vi "解析表格数据.vi"(0 "点位信息表":string[][](table)=[["PCB1-拍照点1(Mark1)", "-73.376", "-164.238", "0.000", "-103.848", "565.620", "384.924", "377.049", "0.000", "0.000", "0.000", "0", "8", "94", "1"], ["PCB1-拍照点2(Mark2)", "-260.376", "-49.239", "0.000", "-290.450", "681.264", "384.924", "377.049", "0.000", "0.000", "0.000", "-180", "8", "94", "1"], ["拍照点3", "-73.376", "-49.239", "0.000", "-103.451", "680.618", "384.924", "377.049", "0.000", "0.000", "0.000", "0", "8", "94", "1"], ["拍照点4", "-260.376", "-164.238", "0.000", "-290.847", "566.266", "384.924", "377.049", "0.000", "0.000", "0.000", "-180", "8", "94", "1"], ["拍照点5", "-260.376", "-104.239", "0.000", "-290.640", "626.265", "384.924", "377.049", "0.000", "0.000", "0.000", "-180", "8", "94", "1"], ["拍照点6", "-240.876", "-23.738", "0.000", "-270.862", "706.698", "384.924", "377.049", "0.000", "0.000", "0.000", "90", "8", "94", "1"], ["拍照点7", "-190.876", "-23.738", "0.000", "-220.862", "706.525", "384.924", "377.049", "0.000", "0.000", "0.000", "90", "8", "94", "0"], ["拍照点8", "-142.876", "-23.738", "0.000", "-172.862", "706.359", "384.924", "377.049", "0.000", "0.000", "0.000", "90", "8", "94", "0"], ["拍照点9", "-92.876", "-23.738", "0.000", "-122.863", "706.187", "384.924", "377.049", "0.000", "0.000", "0.000", "90", "8", "94", "0"], ["拍照点10", "-73.376", "-104.239", "0.000", "-103.641", "625.619", "384.924", "377.049", "0.000", "0.000", "0.000", "0", "8", "94", "0"], ["拍照点11", "-112.876", "-169.238", "0.000", "-143.365", "560.756", "384.924", "377.049", "0.000", "0.000", "0.000", "-90", "8", "94", "0"], ["拍照点12", "-220.876", "-169.238", "0.000", "-251.364", "561.130", "384.924", "377.049", "0.000", "0.000", "0.000", "0", "8", "94", "0"], ["PCB2-拍照点1(Mark3)", "-73.376", "-164.238", "0.000", "151.457", "565.201", "384.924", "377.049", "0.000", "0.000", "-3.000", "0", "8", "94", "1"], ["PCB2-拍照点2(Mark4)", "-260.376", "-49.239", "0.000", "-35.509", "680.255", "384.924", "377.049", "0.000", "0.000", "-3.000", "-180", "8", "94", "1"], ["拍照点3", "-73.376", "-49.239", "0.000", "151.491", "680.200", "384.924", "377.049", "0.000", "0.000", "-3.000", "0", "8", "94", "1"], ["拍照点4", "-260.376", "-164.238", "0.000", "-35.543", "565.256", "384.924", "377.049", "0.000", "0.000", "-3.000", "-180", "8", "94", "1"], ["拍照点5", "-260.376", "-104.239", "0.000", "-35.525", "625.255", "384.924", "377.049", "0.000", "0.000", "-3.000", "-180", "8", "94", "1"], ["拍照点6", "-240.876", "-23.738", "0.000", "-16.001", "705.751", "384.924", "377.049", "0.000", "0.000", "-3.000", "90", "8", "94", "1"], ["拍照点7", "-190.876", "-23.738", "0.000", "33.999", "705.736", "384.924", "377.049", "0.000", "0.000", "0.000", "90", "8", "94", "0"], ["拍照点8", "-142.876", "-23.738", "0.000", "81.999", "705.722", "384.924", "377.049", "0.000", "0.000", "0.000", "90", "8", "94", "0"], ["拍照点9", "-92.876", "-23.738", "0.000", "131.999", "705.707", "384.924", "377.049", "0.000", "0.000", "0.000", "90", "8", "94", "0"], ["拍照点10", "-73.376", "-104.239", "0.000", "151.475", "625.200", "384.924", "377.049", "0.000", "0.000", "0.000", "0", "8", "94", "0"], ["拍照点11", "-112.876", "-169.238", "0.000", "111.956", "560.213", "384.924", "377.049", "0.000", "0.000", "0.000", "-90", "8", "94", "0"], ["拍照点12", "-220.876", "-169.238", "0.000", "3.956", "560.245", "384.924", "377.049", "0.000", "0.000", "0.000", "0", "8", "94", "0"]]) -> (4 "基本信息":T2, 6 "布线前甩线":string[][](table), 8 "布线点位":string[][](table), 10 "布线后甩线":string[][](table), 15 "进出线编码":cluster{"进线编码":i32, "出线编码":i32}[](array[cluster]))   [LabVIEW 2014]
uses:
  Global.vi
panel:
  out "当前线号布线轨迹示意图":T1(plugin-control)
  out "甩线后":dbl[](array[numeric])
  out "布线":dbl[](array[numeric])
  out "甩线前":dbl[](array[numeric])
  out "线号ok":bool
  out "数据正常":bool
  in  "基本信息":T2
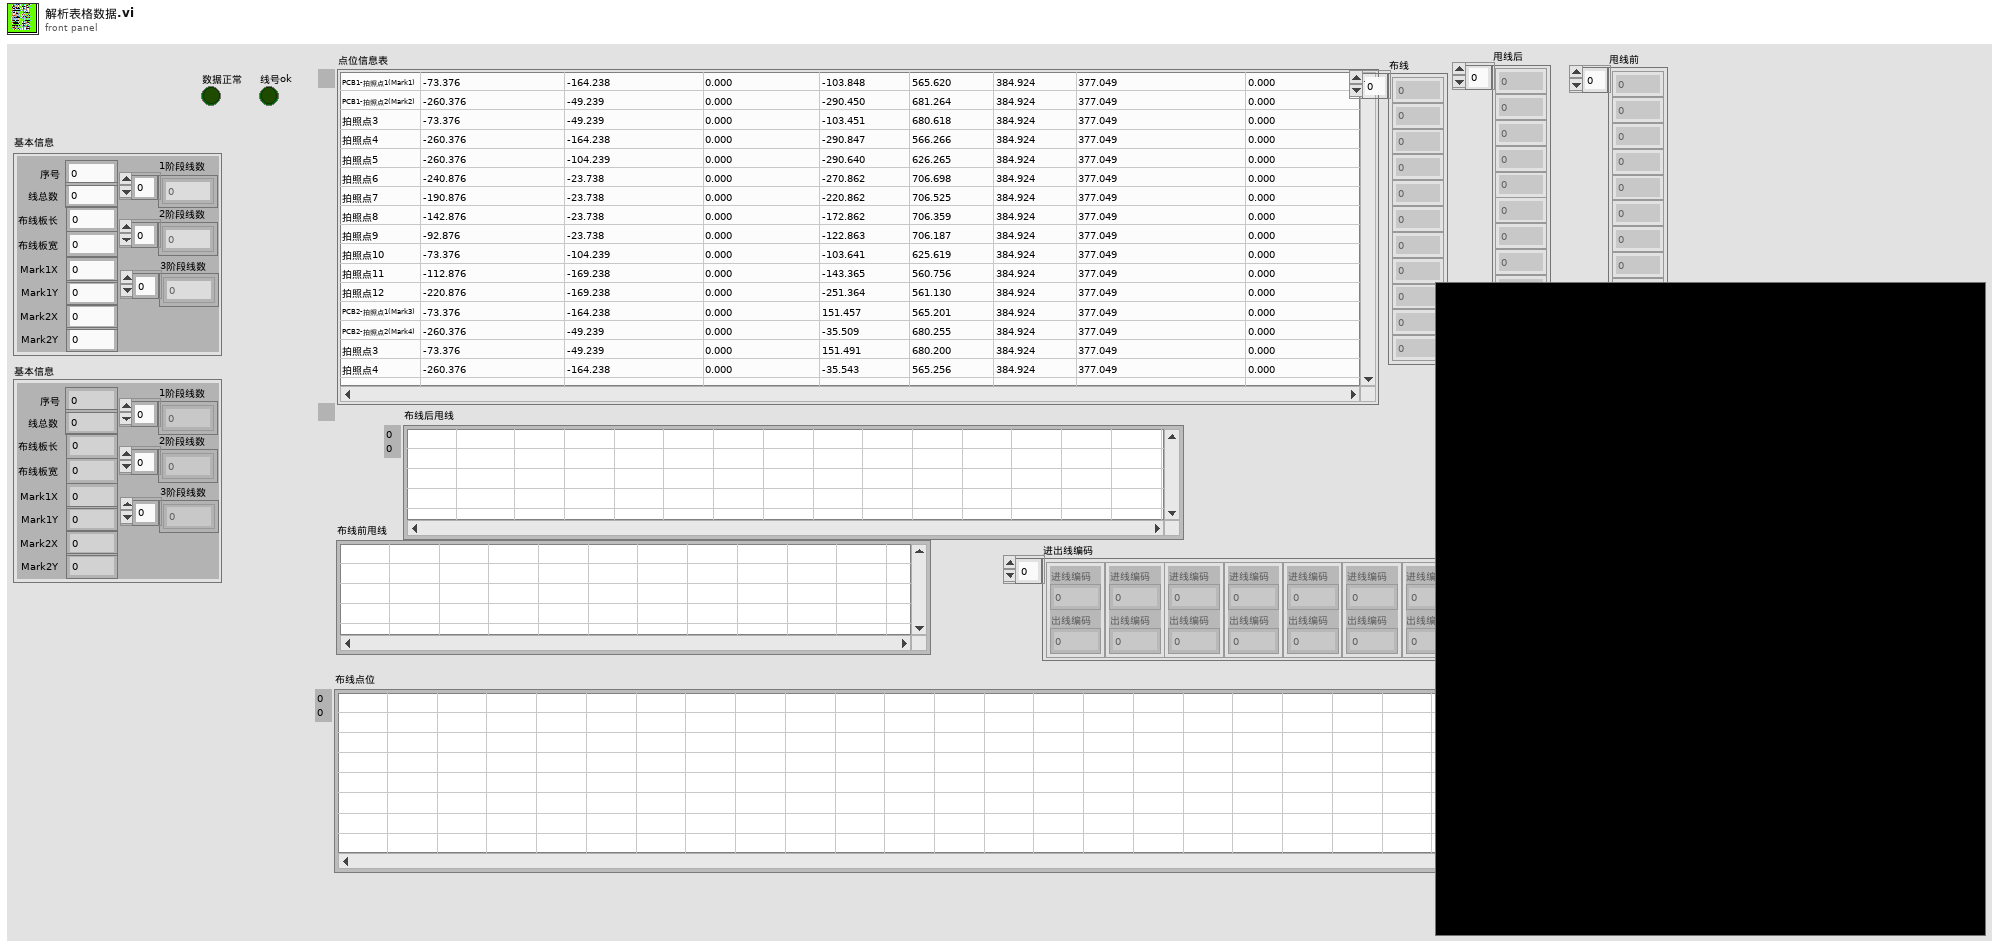
[diagram p1: front panel]
types:
  T1 = typedef "IMAQ Image.ctl" = refnum<image>
  T2 = typedef "基本信息.ctl" = cluster{"序号":dbl, "线总数":dbl, "布线板长":dbl, "布线板宽":dbl, "Mark1X":dbl, "Mark1Y":dbl, "Mark2X":dbl, "Mark2Y":dbl, "1阶段线数":dbl[], "2阶段线数":dbl[], "3阶段线数":dbl[]}
  T3 = typedef "XYPos.ctl" = cluster{"X":dbl, "Y":dbl}
  T4 = typedef "mark规格.ctl" = cluster{"X下限":dbl, "X上限":dbl, "Y下限":dbl, "Y 上限":dbl, "angle下限":dbl, "angle上限":dbl}
  T5 = cluster{"甩线补偿值":cluster{"下边":dbl, "距离上边":dbl, "左边":dbl, "右边":dbl}, "补偿甩线坐标偏移":T3, "mark点模组补偿":T3, "出线补偿值":dbl, "mark规格":T4}
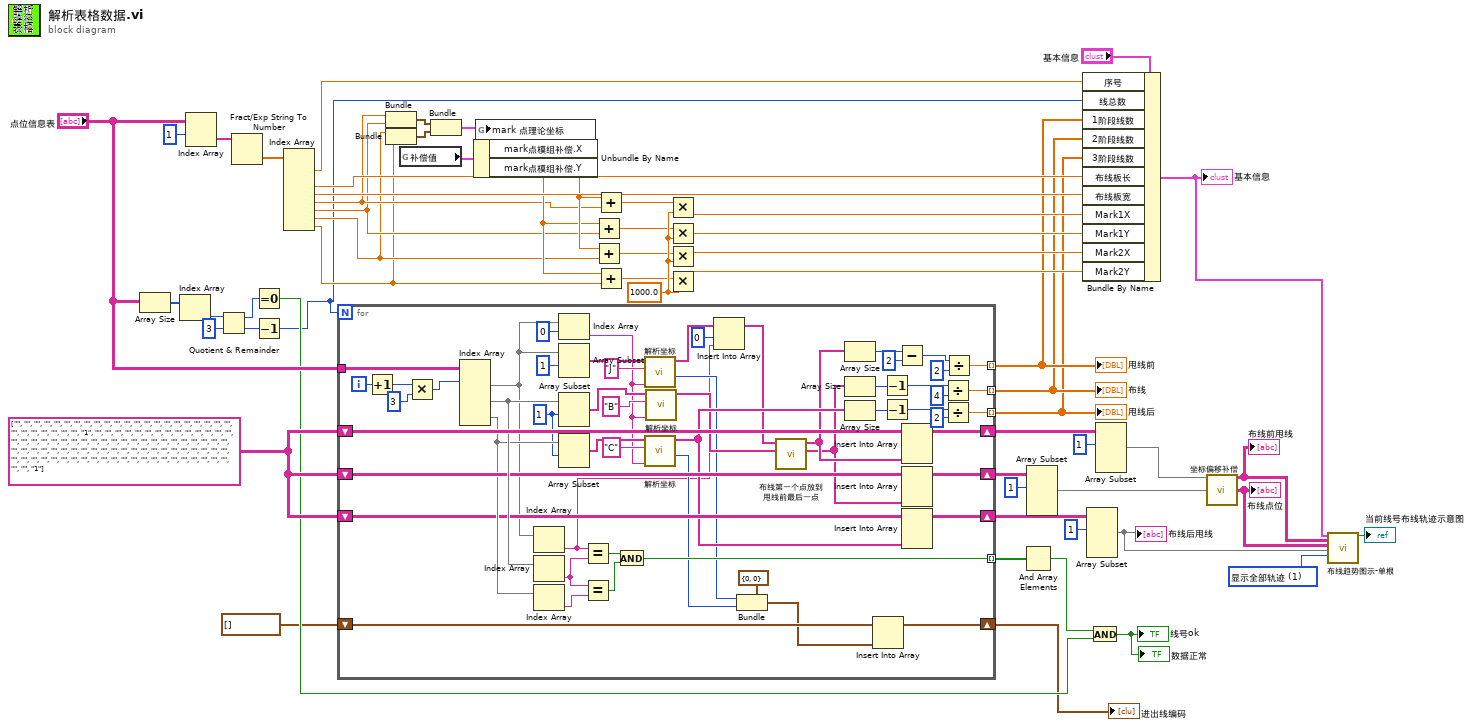
[diagram p0: block diagram]
diagram:
  w3 = u16 1 items=["显示单根轨迹", "显示全部轨迹"] ("轨迹选择")
  w23 = 1000.0 ("y")
  w50 = string[][] [["", "", "", "", "", "", "", "", "", "", "", "", "", "", "", "", "", "", "", "", "", "", "", "", "", "", "", "", "", "1", "", "", "", "", "", "", "", "", "", "", "", "", "", "", "", "", "", "", "", "", "", "", "", "", "", "", "", "", "", "", "", "", "", "", "", "", "", "", "", "", "", "", "", "", "", "", "", "", "", "", "", "", "", "", "", "", "", "", "", "", "", "", "", "", "", "", "", "", "", "", "", "", "", "", "", "", "", "", "", "", "", "", "1"]]
  n1 = Array Size(array="点位信息表") -> (size(s)=w54:i32[])
  n2 = Index Array(array=w54) -> (element=w53:i32)  [unwired: 1 in]
  n3 = Index Array(array="点位信息表", index (row)=1 ("索引 (行)")) -> (element=w56:string[])  [unwired: 1 in]
  n4 = Quotient & Remainder(x=w53, y=3) -> (x-y*floor(x/y)=w51:i32, floor(x/y)=w48:i32)
  n5 = Fract/Exp String To Number(string=w56) -> (number=w47:dbl[])  [unwired: 3 in, 1 out]
  n6 = Equal To 0?(x=w51) -> (x = 0?=w38:bool)
  n7 = Decrement(x=w48) -> (x-1=w8:i32)
  n8 = Index Array(array=w47) -> (element #1=w33:dbl, element #3=w46:dbl, element #4=w45:dbl, element #5=w16:dbl, element #6=w15:dbl, element #7=w11:dbl, element #8=w10:dbl)  [unwired: 8 in, 1 out]
  n9 = for {
    N: w8 -> [_]
    tunnel: "点位信息表" -> [w113]
    tunnel: [w104] -> w40 mode=indexing
    shift-right: [w100] -> w32
    shift-left: w50 -> [w103]
    shift-right: [w91] -> w27
    shift-left: w50 -> [w96]
    shift-right: [w90] -> w28
    shift-left: w50 -> [w89]
    tunnel: [w87] -> w36 mode=indexing
    tunnel: [w83] -> w35 mode=indexing
    tunnel: [w82] -> w34 mode=indexing
    shift-right: [w69] -> w24
    shift-left: cluster{"进线编码":i32, "出线编码":i32}[] [] -> [w71]
    i -> [w112]
    w75 = 1 ("索引")
    n10 = Increment(x=w112) -> (x+1=w109:i32)
    n11 = Multiply(x=w109, y=3) -> (x*y=w110:i32)
    n12 = Index Array(array=w113, index (row) #1=w110) -> (element #1=w78:string[], element #2=w99:string[], element #3=w94:string[])  [unwired: 5 in]
    n13 = Index Array(array=w78) -> (element=w62:string)  [unwired: 1 in]
    n14 = Index Array(array=w99) -> (element=w108:string)  [unwired: 1 in]
    n15 = Index Array(array=w94) -> (element=w107:string)  [unwired: 1 in]
    n16 = Index Array(array=w78, index=0 ("索引")) -> (element=w76:string)
    n17 = Array Subset(array=w78, index=1 ("索引")) -> (w102:string[])  [unwired: 1 in]
    n18 = Array Subset(array=w99, index=w75) -> (w97:string[])  [unwired: 1 in]
    n19 = Array Subset(array=w94, index=w75) -> (w93:string[])  [unwired: 1 in]
    n20 = Equal?(x=w62, y=w108) -> (x = y?=w106:bool)
    n21 = Equal?(x=w108, y=w107) -> (x = y?=w105:bool)
    n22 = And(x=w106, y=w105) -> (x .and. y?=w104:bool)
    n23 = call "解析坐标.vi"("线号"=w76, "匹配字符"="J", "解析数组"=w102) -> ("编码数值"=w74:i32, "坐标xy顺序"=w64:string[])  [unwired: 6 in, 1 out]
    n24 = call "解析坐标.vi"("线号"=w76, "匹配字符"="C", "解析数组"=w93) -> ("编码数值"=w73:i32, "坐标xy顺序"=w85:string[])  [unwired: 6 in, 1 out]
    n25 = call "解析坐标.vi"("线号"=w76, "匹配字符"="B", "解析数组"=w97) -> ("坐标xy顺序"=w81:string[])  [unwired: 6 in, 2 out]
    n26 = Insert Into Array(array=w64, index=0 ("索引"), new element=w62) -> (w63:string[])
    n27 = Bundle(cluster=cluster{"进线编码":i32, "出线编码":i32} {"进线编码"=0, "出线编码"=0}, "进线编码"=w74, "出线编码"=w73) -> (w70:cluster{"进线编码":i32, "出线编码":i32})
    n28 = call "布线第一个点放到甩线前最后一点.vi"("布线点"=w81, "甩线前"=w63) -> ("布线点 2"=w79:string[], "甩线前 2"=w80:string[])  [unwired: 8 in]
    n29 = Array Size(array=w80) -> (size(s)=w68:i32)
    n30 = Array Size(array=w79) -> (size(s)=w61:i32)
    n31 = Array Size(array=w85) -> (size(s)=w59:i32)
    n32 = Insert Into Array(array=w71, new element=w70) -> (w69:cluster{"进线编码":i32, "出线编码":i32}[])  [unwired: 1 in]
    n33 = Decrement(x=w61) -> (x-1=w60:i32)
    n34 = Decrement(x=w59) -> (x-1=w58:i32)
    n35 = Subtract(x=w68, y=2) -> (x-y=w67:i32)
    n36 = Insert Into Array(array=w103, new element=w80) -> (w100:string[][])  [unwired: 2 in]
    n37 = Insert Into Array(array=w96, new element=w79) -> (w91:string[][])  [unwired: 2 in]
    n38 = Insert Into Array(array=w89, new element=w85) -> (w90:string[][])  [unwired: 2 in]
    n39 = Divide(x=w60, y=4) -> (x/y=w83:dbl)
    n40 = Divide(x=w58, y=2) -> (x/y=w82:dbl)
    n41 = Divide(x=w67, y=2) -> (x/y=w87:dbl)
  }
  "甩线前" <- w36
  "布线" <- w35
  "甩线后" <- w34
  "进出线编码" <- w24
  n42 = Bundle(w16, w15) -> (w13:cluster{dbl, dbl})  [unwired: 1 in]
  n43 = Bundle(w11, w10) -> (w12:cluster{dbl, dbl})  [unwired: 1 in]
  n44 = global read "Global.vi" "补偿值"() -> (w7:T5)
  n45 = Bundle(w13, w12) -> (w14:cluster{cluster{dbl, dbl}, cluster{dbl, dbl}})  [unwired: 1 in]
  n46 = Unbundle By Name(w7) -> ("mark点模组补偿.X"=w19:dbl, "mark点模组补偿.Y"=w17:dbl)
  n47 = global write "Global.vi" "mark 点理论坐标"(w14) -> ()
  n48 = Add(x=w17, y=w15) -> (x+y=w21:dbl)
  n49 = Add(x=w19, y=w11) -> (x+y=w20:dbl)
  n50 = Add(x=w19, y=w16) -> (x+y=w22:dbl)
  n51 = Add(x=w17, y=w10) -> (x+y=w18:dbl)
  n52 = Multiply(x=w22, y=w23) -> (x*y=w44:dbl)
  n53 = Multiply(x=w21, y=w23) -> (x*y=w43:dbl)
  n54 = Multiply(x=w20, y=w23) -> (x*y=w42:dbl)
  n55 = Multiply(x=w18, y=w23) -> (x*y=w41:dbl)
  n56 = And Array Elements(Boolean array=w40) -> (logical AND=w39:bool)
  n57 = Array Subset(array=w27, index (row)=1 ("索引")) -> (w26:string[][])  [unwired: 3 in]
  n58 = Bundle By Name(cluster="基本信息", "序号"=w33, "线总数"=w8, "1阶段线数"=w36, "2阶段线数"=w35, "3阶段线数"=w34, "布线板长"=w46, "布线板宽"=w45, "Mark1X"=w44, "Mark1Y"=w43, "Mark2X"=w42, "Mark2Y"=w41) -> (w2:T2)
  "基本信息" <- w2
  n59 = Array Subset(array=w28, index (row)=1 ("索引")) -> (w1:string[][])  [unwired: 3 in]
  "布线后甩线" <- w1
  n60 = And(x=w39, y=w38) -> (x .and. y?=→"数据正常" →"线号ok":bool)
  n61 = Array Subset(array=w32, index (row)=1 ("索引")) -> (w9:string[][])  [unwired: 3 in]
  n62 = call "坐标偏移补偿.vi"("布线前甩线"=w9, "布线点位"=w26) -> ("布线前甩线矫正后"=w5:string[][], "布线点矫正后"=w4:string[][])  [unwired: 11 in, 1 out]
  "布线前甩线" <- w5
  "布线点位" <- w4
  n63 = call "布线趋势图示-单根.vi"("基本信息"=w2, "布线前甩线"=w5, "布线点位"=w4, "布线后甩线"=w1, "轨迹选择"=w3) -> ("引用句柄输出"=→"当前线号布线轨迹示意图":T1)  [unwired: 14 in]
